vi "Run.vi"(8 "error in (no error)":errorcluster caption="entrée d'erreur (pas d'erreur)", 9 "y_prob":string[][](array[string]), 10 "y_true":string[][](array[string]), 11 "Brier_Score_Loss.lvclass":refnum<class "Brier_Score_Loss.lvclass">) -> (0 "error out":errorcluster caption="sortie d'erreur", 2 "Score":string, 3 "Brier_Score_Loss.lvclass":refnum<class "Brier_Score_Loss.lvclass">)   [LabVIEW 2020, in "Brier_Score_Loss.lvclass"]
doc: "Returns :\n\n- score : float\nBrier score"
uses:
  Brier_Score_Loss.lvclass
  Brier_Score_Loss.lvclass/Brier_Score_Loss.ctl
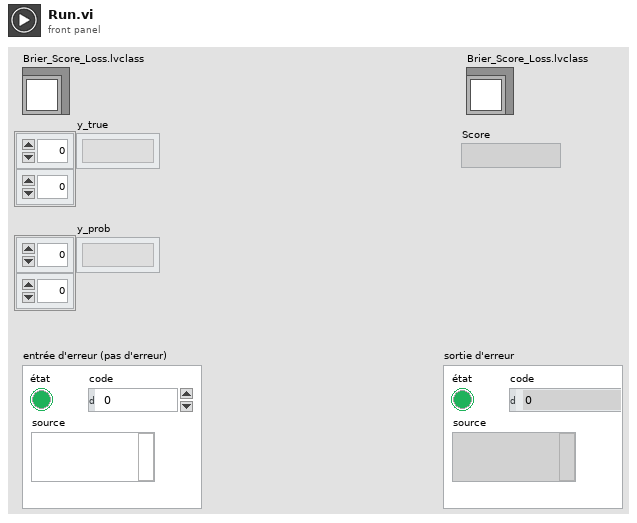
[diagram p1: front panel]
types:
  T1 = cluster{"dtype_pos_label":string, "pos_label":string}
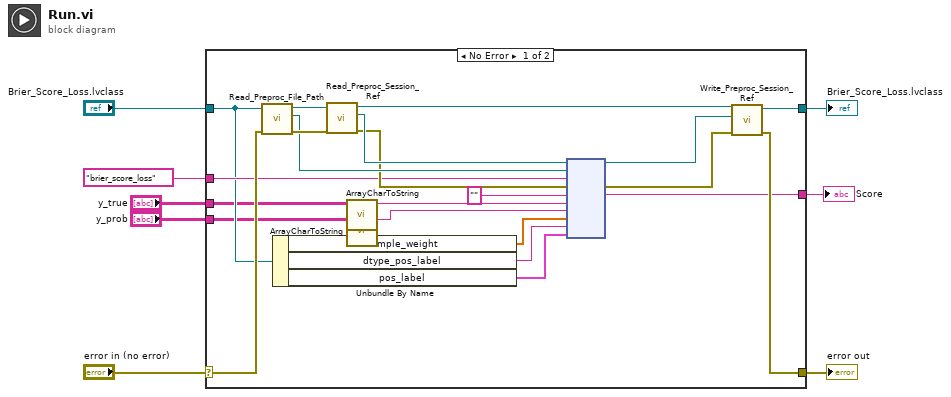
[diagram p0: block diagram]
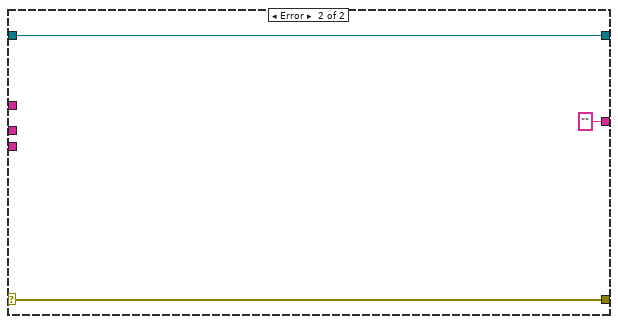
[diagram p2: hidden frame]
diagram:
  n1 = case shown="No Error" "error in (no error)" {
    selector: "error in (no error)" -> [w19 w33]
    tunnel: [w20 w33] -> w7
    tunnel: [w21 w32] -> w5
    tunnel: "Brier_Score_Loss.lvclass" -> [w16 w32]
    tunnel: "brier_score_loss" -> [w18 _]
    tunnel: [w17 ""] -> w4
    tunnel: "y_true" -> [w12 _]
    tunnel: "y_prob" -> [w10 _]
    frame No Error {
      n2 = call-dynamic "Read_Preproc_File_Path.vi"("error in (no error)"=w19, "Python in"=w16) -> ("error out"=w29:errorcluster, "File_Path"=w28:path, "Python out"=w30:refnum<class "Brier_Score_Loss.lvclass">)  [unwired: 7 in]
      n3 = Unbundle By Name(w16) -> ("sample_weight"=w15:dbl[], "dtype_pos_label"=w14:string, "pos_label"=w13:T1)
      n4 = call-dynamic "Read_Preproc_Session_Ref.vi"("error in (no error)"=w29, "Python in"=w30) -> ("error out"=w26:errorcluster, "Session_ref"=w27:refnum<k35>, "Python out"=w25:refnum<class "Brier_Score_Loss.lvclass">)  [unwired: 7 in]
      n5 = call "ArrayCharToString.vi"("TAB"=w12) -> ("Instruction"=w11:string)  [unwired: 10 in]
      n6 = call "ArrayCharToString.vi"("TAB"=w10) -> ("Instruction"=w9:string)  [unwired: 10 in]
      n7 = node(w27, w28, w18, w26, "", w11, w9, w15, w14, w13) -> (w23:refnum<k35>, w24:errorcluster, w17:string)  [unwired: 5 in, 2 out]
      n8 = call-dynamic "Write_Preproc_Session_Ref.vi"("error in (no error)"=w24, "Session_ref"=w23, "Python in"=w25) -> ("error out"=w20:errorcluster, "Python out"=w21:refnum<class "Brier_Score_Loss.lvclass">)  [unwired: 7 in]
    }
    frame Error {
    }
  }
  "error out" <- w7
  "Brier_Score_Loss.lvclass" <- w5
  "Score" <- w4
